vi "Stop watch.vi"() -> ()   [LabVIEW 2010]
panel:
  in  "Stop":bool caption="(F2)"
  out "Elapsed Time":dbl[unit] format="%<%H:%M:%S%3u>t"
  out "Flow rate":dbl[unit]
  in  "Volume measured":dbl[unit]
  in  "Quit":bool
  in  "Start":bool caption="(F1)"
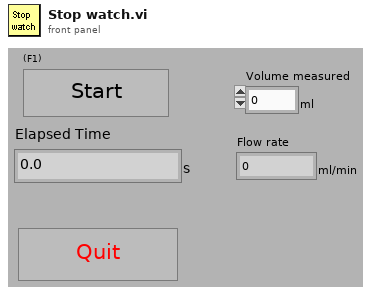
[diagram p1: front panel]
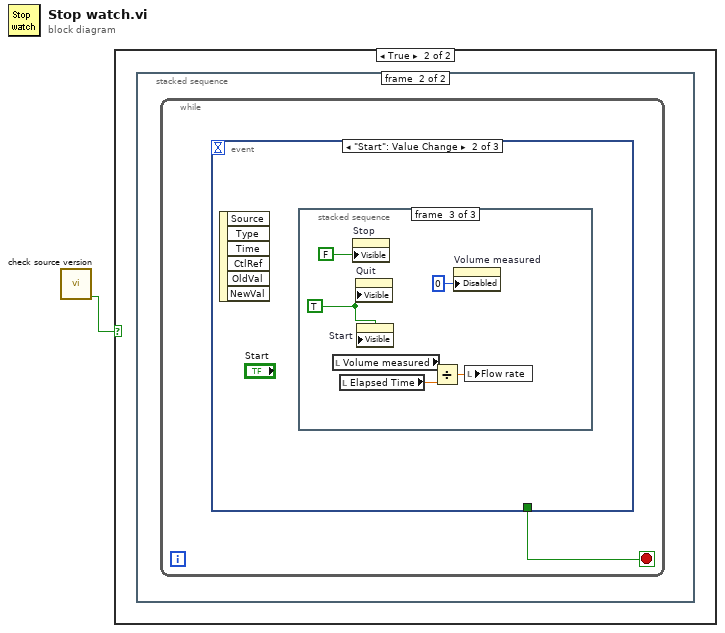
[diagram p0: block diagram]
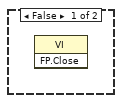
[diagram p2: hidden frame]
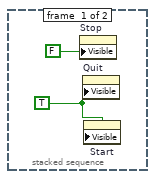
[diagram p3: hidden frame]
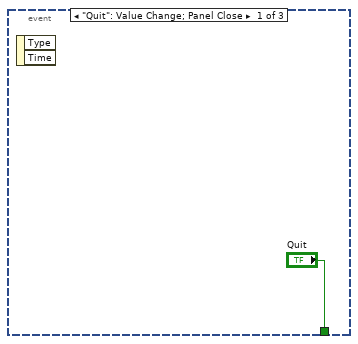
[diagram p4: hidden frame]
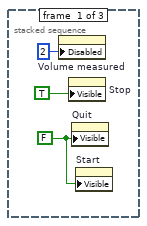
[diagram p5: hidden frame]
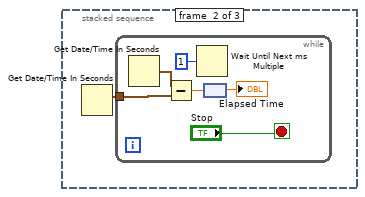
[diagram p6: hidden frame]
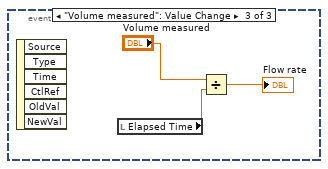
[diagram p7: hidden frame]
diagram:
  n1 = call "check source version.vi"() -> ("continue running?"=w1:bool)  [unwired: 2 in, 3 out]
  n2 = case shown="True" w1 {
    frame False {
      n3 = invoke class="VI" method="FP.Close"() -> ()  [unwired: 3 in, 3 out]
    }
    frame True {
      n4 = stacked-sequence {
        frame #0 {
          w2 = TRUE ("Visible")
          n5 = property on="Stop" class="Bool"("Visible"=FALSE) -> ()  [unwired: 2 in, 2 out]
          n6 = property on="Quit" class="Bool"("Visible"=w2) -> ()  [unwired: 2 in, 2 out]
          n7 = property on="Start" class="Bool"("Visible"=w2) -> ()  [unwired: 2 in, 2 out]
        }
        frame #1 {
          n8 = while {
            stop <- w4 stop-if-true
            n9 = event shown="[1] \"Start\": Value Change" {
              selector: _ -> [_ _ _]
              dyn-events: _ -> [_ _ _]
              timeout: _ -> [_ _ _]
              tunnel: ["Quit" _ _] -> w4
              event "Quit": Value Change; Panel Close {
                n10 = event-data() -> ()  [unwired: 1 in, 2 out]
              }
              event "Start": Value Change {
                n11 = event-data() -> ()  [unwired: 1 in, 6 out]
                n12 = stacked-sequence {
                  frame #0 {
                    w7 = FALSE ("Visible")
                    n13 = property on="Volume measured" class="DigNum (strict)"("Disabled"=u8 2) -> ()  [unwired: 2 in, 2 out]
                    n14 = property on="Stop" class="Bool"("Visible"=TRUE) -> ()  [unwired: 2 in, 2 out]
                    n15 = property on="Quit" class="Bool"("Visible"=w7) -> ()  [unwired: 2 in, 2 out]
                    n16 = property on="Start" class="Bool"("Visible"=w7) -> ()  [unwired: 2 in, 2 out]
                  }
                  frame #1 {
                    n17 = Get Date/Time In Seconds() -> (seconds since 1Jan1904=w9:timestamp)
                    n18 = while {
                      tunnel: w9 -> [w14]
                      stop <- "Stop" stop-if-true
                      n19 = Get Date/Time In Seconds() -> (seconds since 1Jan1904=w15:timestamp)
                      n20 = Subtract(x=w15, y=w14) -> (x-y=w11:dbl)
                      n21 = Wait Until Next ms Multiple(millisecond multiple=u32 1) -> ()  [unwired: 1 out]
                      n22 = node(w11) -> (→"Elapsed Time":dbl[unit])
                    }
                  }
                  frame #2 {
                    w17 = TRUE ("Visible")
                    n23 = local read "Volume measured"() -> (w19:dbl[unit])
                    n24 = local read "Elapsed Time"() -> (w20:dbl[unit])
                    n25 = property on="Stop" class="Bool"("Visible"=FALSE) -> ()  [unwired: 2 in, 2 out]
                    n26 = property on="Quit" class="Bool"("Visible"=w17) -> ()  [unwired: 2 in, 2 out]
                    n27 = property on="Start" class="Bool"("Visible"=w17) -> ()  [unwired: 2 in, 2 out]
                    n28 = Divide(x=w19, y=w20) -> (x/y=w18:dbl[unit])
                    n29 = property on="Volume measured" class="DigNum (strict)"("Disabled"=u8 0) -> ()  [unwired: 2 in, 2 out]
                    n30 = local write "Flow rate"(w18) -> ()
                  }
                }
              }
              event "Volume measured": Value Change {
                n31 = event-data() -> ()  [unwired: 1 in, 6 out]
                n32 = local read "Elapsed Time"() -> (w23:dbl[unit])
                n33 = Divide(x="Volume measured", y=w23) -> (x/y=→"Flow rate":dbl[unit])
              }
            }
          }
        }
      }
    }
  }
